vi "Configure Measurement Characteristics (FFT).vi"(0 "VISA resource name":refnum<visa-resource-name>, 5 "Peak Level (-40.0 dB)":dbl, 7 "1st Peak Number (1)":i32, 9 "2nd Peak Number (1)":i32, 11 "error in (no error)":errorcluster) -> (4 "VISA resource name out":refnum<visa-resource-name>, 15 "error out":errorcluster)   [LabVIEW 2009, in "Agilent 8000 Series.lvlib"]
doc: "Sets the peak search threshold value, the first peak number and second peak number for FFT measurements. \n\nThe first peak number and second peak number are used for measurement of FFT delta frequency and FFT delta magnitude."
uses:
  Agilent 8000 Series.lvlib
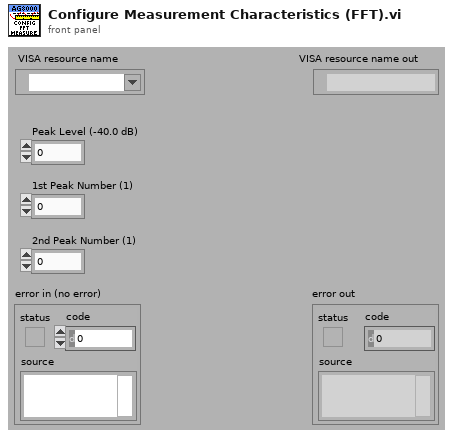
[diagram p1: front panel]
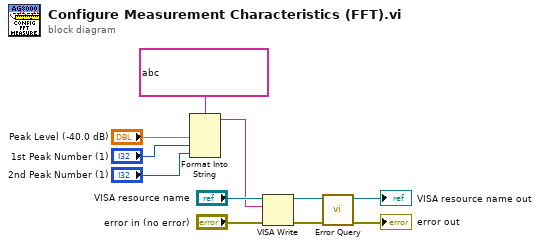
[diagram p0: block diagram]
diagram:
  n1 = Format Into String(format string=string ?, "Peak Level (-40.0 dB)", "1st Peak Number (1)", "2nd Peak Number (1)") -> (resulting string=w1:string)  [unwired: 2 in, 1 out]
  n2 = VISA Write(VISA resource name="VISA resource name", write buffer=w1, error in (no error)="error in (no error)") -> (VISA resource name out=w7:refnum<visa-resource-name>, error out=w6:errorcluster)  [unwired: 1 out]
  n3 = call "Error Query.vi"("error in (no error)"=w6, "VISA resource name"=w7) -> ("error out"=→"error out":errorcluster, "VISA resource name out"=→"VISA resource name out":refnum<visa-resource-name>)  [unwired: 6 in, 2 out]
